vi "Correction.vi"(0 "Calibrated Image":T1(plugin-control), 5 "Vertical/Horizontal":enum16{"Horizontal", "Vertical"}(ring), 7 "Algo Type":string, 9 "appended array":cluster{"X":sgl, "Y":sgl}[][](array[cluster]), 11 "error in (no error)":errorcluster) -> (4 "Mesurement Value":sgl, 6 "Array":sgl[](array[numeric]), 15 "error IO":errorcluster)   [LabVIEW 2019, in "Algorithm.lvclass"]
uses:
  FrameworkOverrides/Algorithm.lvclass
  <vilib>/vision/NI_Vision_Development_Module.lvlib
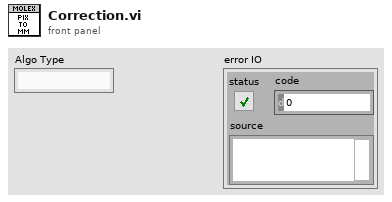
[diagram p1: front panel]
types:
  T1 = typedef "IMAQ Image.ctl" = refnum<image>
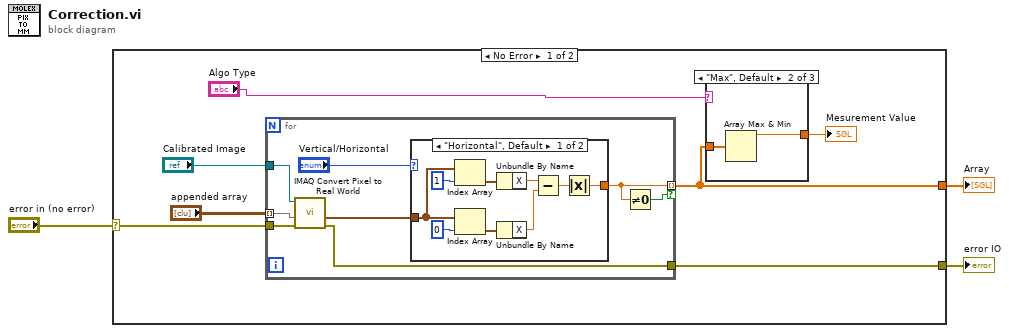
[diagram p0: block diagram]
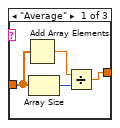
[diagram p2: hidden frame]
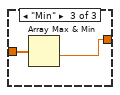
[diagram p3: hidden frame]
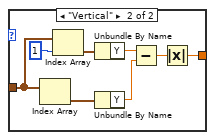
[diagram p4: hidden frame]
diagram:
  n1 = case shown="No Error" "error in (no error)" {
    selector: "error in (no error)" -> [w8 w44]
    tunnel: [w7 w44] -> w2
    tunnel: [w5 _] -> w1
    frame No Error {
      n2 = for {
        tunnel: "appended array" -> [w26] mode=indexing
        tunnel: "Calibrated Image" -> [w25]
        tunnel: [w19] -> w5 mode=indexing if=w20
        tunnel: w8 -> [w22]
        tunnel: [w21] -> w7
        n3 = call "IMAQ Convert Pixel to Real World"("error in (no error)"=w22, "Array of Pixel Coordinates"=w26, "Calibrated Image"=w25) -> ("error out"=w21:errorcluster, "Array of Real World Coordinates"=w24:cluster{"X":sgl, "Y":sgl}[])  [unwired: 3 in, 4 out]
        n4 = case shown="\"Horizontal\", Default" "Vertical/Horizontal" {
          tunnel: w24 -> [w30 w43]
          tunnel: [w27 w36] -> w19
          frame "Horizontal", Default {
            n5 = Index Array(array=w30, index=1) -> (element=w32:cluster{"X":sgl, "Y":sgl})
            n6 = Index Array(array=w30, index=0) -> (element=w34:cluster{"X":sgl, "Y":sgl})
            n7 = Unbundle By Name(w32) -> ("X"=w31:sgl)
            n8 = Unbundle By Name(w34) -> ("X"=w33:sgl)
            n9 = Subtract(x=w31, y=w33) -> (x-y=w29:sgl)
            n10 = Absolute Value(x=w29) -> (abs(x)=w27:sgl)
          }
          frame "Vertical" {
            n11 = Index Array(array=w43) -> (element=w42:cluster{"X":sgl, "Y":sgl})  [unwired: 1 in]
            n12 = Index Array(array=w43, index=1) -> (element=w40:cluster{"X":sgl, "Y":sgl})
            n13 = Unbundle By Name(w40) -> ("Y"=w39:sgl)
            n14 = Unbundle By Name(w42) -> ("Y"=w41:sgl)
            n15 = Subtract(x=w39, y=w41) -> (x-y=w37:sgl)
            n16 = Absolute Value(x=w37) -> (abs(x)=w36:sgl)
          }
        }
        n17 = Not Equal To 0?(x=w19) -> (x != 0?=w20:bool)
      }
      n18 = case shown="\"Max\", Default" "Algo Type" {
        tunnel: w5 -> [w14 w16 w18]
        tunnel: [w11 w15 w17] -> w9
        frame "Average" {
          n19 = Add Array Elements(numeric array=w14) -> (sum=w13:sgl)
          n20 = Array Size(array=w14) -> (size(s)=w12:i32)
          n21 = Divide(x=w13, y=w12) -> (x/y=w11:sgl)
        }
        frame "Max", Default {
          n22 = Array Max & Min(array=w16) -> (max value=w15:sgl)  [unwired: 3 out]
        }
        frame "Min" {
          n23 = Array Max & Min(array=w18) -> (min value=w17:sgl)  [unwired: 3 out]
        }
      }
      "Mesurement Value" <- w9
    }
    frame Error {
    }
  }
  "error IO" <- w2
  "Array" <- w1
